vi "DriveModuleOpen.vi"(6 "Magnet Offset (Degrees)":dbl, 7 "ModualNamePrefix":string, 8 "error in":errorcluster, 9 "EncoderCanID":u8, 10 "SpinCanID":u8, 11 "TravelCanID":u8) -> (0 "error out":errorcluster)   [LabVIEW 2023]
uses:
  <vilib>/Rock Robotics/WPI/ThirdParty/REV Robotics/REVLib/Typedef/Spark MAX Idle Mode.ctl
  <vilib>/Rock Robotics/WPI/ThirdParty/REV Robotics/REVLib/SubVI/Public/SPARK Open Brushless.vi
  <vilib>/Rock Robotics/WPI/ThirdParty/REV Robotics/REVLib/SubVI/Public/SPARK Configure Basic Idle Mode.vi
  <vilib>/Rock Robotics/WPI/ThirdParty/REV Robotics/REVLib/SubVI/Public/SPARK Configure Basic Ramp Rate.vi
  <vilib>/Rock Robotics/WPI/ThirdParty/REV Robotics/REVLib/SubVI/Public/SPARK Configure Encoder Conversion Factors.vi
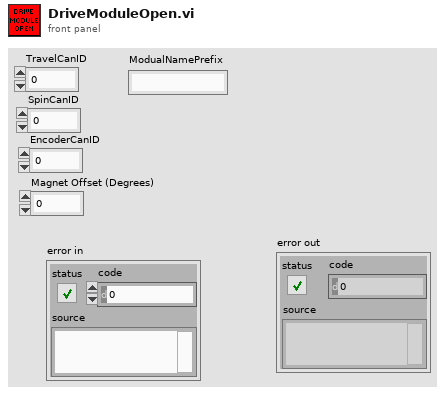
[diagram p1: front panel]
types:
  T1 = cluster{"Future Proof Configs":bool, "MagnetSensorSensorDirection":u16, "MagnetSensorMagnetOffset":dbl, "MagnetSensorAbsoluteSensorDiscontinuityPoint":dbl, "CustomParamsCustomParam0":i16, "CustomParamsCustomParam1":i16}
  T2 = typedef "Spark MAX Idle Mode.ctl" = enum16{"Coast", "Brake"}
  T3 = typedef "WPI_MotorControlDeviceRef.ctl" = cluster{"DeviceStatus":errorcluster, "Type":T4, "PWM":cluster{"PWM Channel":T5, "DeadBand":T6}, "CAN":cluster{"Device Number":u8, "SetOutput VI Ref":variant, "GetOutput VI Ref":variant, "Enable VI Ref":variant, "Disable VI Ref":variant, "Data":variant}, "Invert":bool, "DIO PWM":cluster{"PWM \"Enable\" Channel":T5, "DIOChannel":T7, "PWM Rate":dbl}}
  T4 = typedef "WPI_MotorControlType.ctl" = enum16{"PWM", "CAN", "DIO PWM"}
  T5 = typedef "FPGA_DIOPWMChannel.ctl" = enum8{"PWM 0", "PWM 1", "PWM 2", "PWM 3", "PWM 4", "PWM 5", "PWM 6", "PWM 7", "PWM 8", "PWM 9", "PWM MXP 0", "PWM MXP 1", "PWM MXP 2", "PWM MXP 3", "PWM MXP 4", "PWM MXP 5", "PWM MXP 6", "PWM MXP 7", "PWM MXP 8", "PWM MXP 9", "Invalid"}
  T6 = typedef "WPI_PWMDeadband.ctl" = cluster{"Name":string, "maxPositivePwm":i32, "minPositivePwm":i32, "centerPwm":i32, "maxNegativePwm":i32, "minNegativePwm":i32, "angularRange":u16}
  T7 = typedef "FPGA_DIOChannel.ctl" = enum8{"DIO 0", "DIO 1", "DIO 2", "DIO 3", "DIO 4", "DIO 5", "DIO 6", "DIO 7", "DIO 8", "DIO 9", "DIO MXP 0", "DIO MXP 1", "DIO MXP 2", "DIO MXP 3", "DIO MXP 4", "DIO MXP 5", "DIO MXP 6", "DIO MXP 7", "DIO MXP 8", "DIO MXP 9", "DIO MXP 10", "DIO MXP 11", "DIO MXP 12", "DIO MXP 13", "DIO MXP 14", "DIO MXP 15", "SPI Port CS1", "SPI Port CS2", "SPI Port CS3", "SPI Port MISO", "SPI Port MOSI", "Invalid"}
  T8 = typedef "DeviceReference.ctl" = cluster{"CANbus Name":string, "Device Encoding":u32, "Device Name":string}
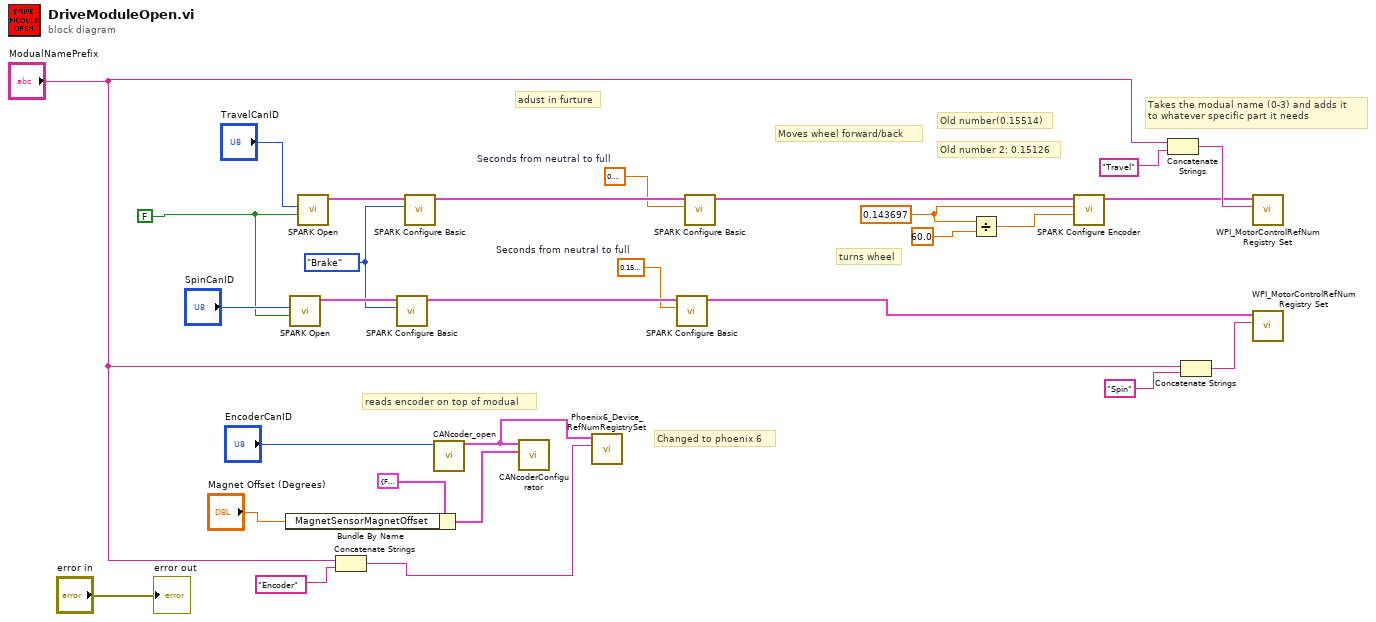
[diagram p0: block diagram]
diagram:
  w7 = sgl 0.15  # Seconds from neutral to full
  w18 = sgl 0.3  # Seconds from neutral to full
  w17 = 0.143697 ("Position Factor (1)")
  w10 = Spark_MAX_Idle_Mode."Brake" ("Idle Mode")
  w12 = FALSE ("Invert")
  # "Changed to phoenix 6"
  # "adust in furture"
  # "Old number 2: 0.15126"
  # "Old number(0.15514)"
  # "reads encoder on top of modual"
  # "turns wheel"
  # "Moves wheel forward/back"
  # "Takes the modual name (0-3) and adds it \nto whatever specific part it needs"
  n1 = Bundle By Name(cluster=T1 {"Future Proof Configs"=FALSE, "MagnetSensorSensorDirection"=0, "MagnetSensorMagnetOffset"=0.0, "MagnetSensorAbsoluteSensorDiscontinuityPoint"=0.5, "CustomParamsCustomParam0"=0, "CustomParamsCustomParam1"=0} ("DeviceConfiguration"), "MagnetSensorMagnetOffset"="Magnet Offset (Degrees)") -> (w4:T1)
  n2 = call-poly <vilib>:"SPARK Open.vi"("Invert"=w12, "Device Number"="SpinCanID") -> ("MotorControlDeviceRef"=w11:T3)  [unwired: 8 in, 1 out]
  n3 = call-poly <vilib>:"SPARK Open.vi"("Invert"=w12, "Device Number"="TravelCanID") -> ("MotorControlDeviceRef"=w20:T3)  [unwired: 8 in, 1 out]
  n4 = Concatenate Strings("ModualNamePrefix", "Encoder" ("refnum name")) -> (w5:string)
  n5 = call-poly <vilib>:"SPARK Configure Basic.vi"("Idle Mode"=w10, "MotorControlDeviceRef in"=w11) -> ("MotorControlDeviceRef out"=w9:T3)  [unwired: 8 in, 1 out]
  n6 = call-poly <vilib>:"SPARK Configure Basic.vi"("Idle Mode"=w10, "MotorControlDeviceRef in"=w20) -> ("MotorControlDeviceRef out"=w19:T3)  [unwired: 8 in, 1 out]
  n7 = call <vilib>:"CANcoder_open.vi"("Device ID"="EncoderCanID") -> ("DeviceReference 2"=w1:T8)  [unwired: 9 in, 1 out]
  n8 = call <vilib>:"CANcoderConfigurator.vi"("DeviceConfiguration"=w4, "DeviceReference"=w1) -> ()  [unwired: 9 in, 1 out]
  n9 = call <vilib>:"Phoenix6_Device_RefNumRegistrySet.vi"("refnum name"=w5, "DeviceReference"=w1) -> ()  [unwired: 8 in, 2 out]
  n10 = call-poly <vilib>:"SPARK Configure Basic.vi"("Seconds from neutral to full (0)"=w7, "MotorControlDeviceRef in"=w9) -> ("MotorControlDeviceRef"=w8:T3)  [unwired: 8 in, 1 out]
  n11 = call-poly <vilib>:"SPARK Configure Basic.vi"("Seconds from neutral to full (0)"=w18, "MotorControlDeviceRef in"=w19) -> ("MotorControlDeviceRef"=w15:T3)  [unwired: 8 in, 1 out]
  n12 = Divide(x=w17, y=60.0) -> (x/y=w16:dbl)
  n13 = call-poly <vilib>:"SPARK Configure Encoder.vi"("Velocity Conversion Factor"=w16, "Position Conversion Factor"=w17, "MotorControlDeviceRef in"=w15) -> ("MotorControlDeviceRef out"=w14:T3)  [unwired: 7 in, 1 out]
  n14 = Concatenate Strings("ModualNamePrefix", "Travel" ("refnum name")) -> (w28:string)
  n15 = Concatenate Strings("ModualNamePrefix", "Spin" ("refnum name")) -> (w26:string)
  n16 = call <vilib>:"WPI_MotorControlRefNum Registry Set.vi"("refnum name"=w28, "MotorControlDevRef"=w14) -> ()  [unwired: 8 in, 2 out]
  n17 = call <vilib>:"WPI_MotorControlRefNum Registry Set.vi"("refnum name"=w26, "MotorControlDevRef"=w8) -> ()  [unwired: 8 in, 2 out]
  "error out" <- "error in"
